vi "distribute_equally.vi"(8 "error in (no error)":errorcluster, 11 "TrajectoryDL091126GenericVoxel in":refnum<class "TrajectoryDL091126GenericVoxel.lvclass">) -> (0 "error out":errorcluster, 2 "failed?":bool, 3 "TrajectoryDL091126GenericVoxel out":refnum<class "TrajectoryDL091126GenericVoxel.lvclass">)   [LabVIEW 2010, in "TrajectoryDL091126GenericVoxel.lvclass"]
uses:
  TrajectoryDL091126GenericVoxel.lvclass
  common/classes/SpaceVector/SpaceVector/SpaceVector.lvclass
  common/classes/ErrorController/ErrorController/class_data.vi
  common/classes/ErrorController/ErrorController/ErrorController.lvclass
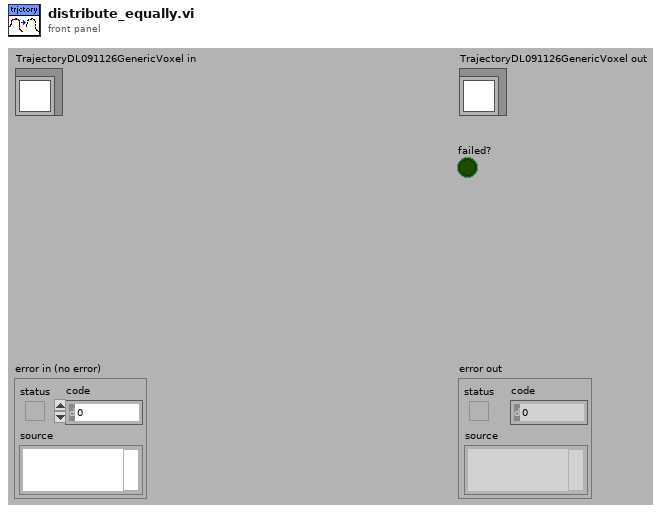
[diagram p1: front panel]
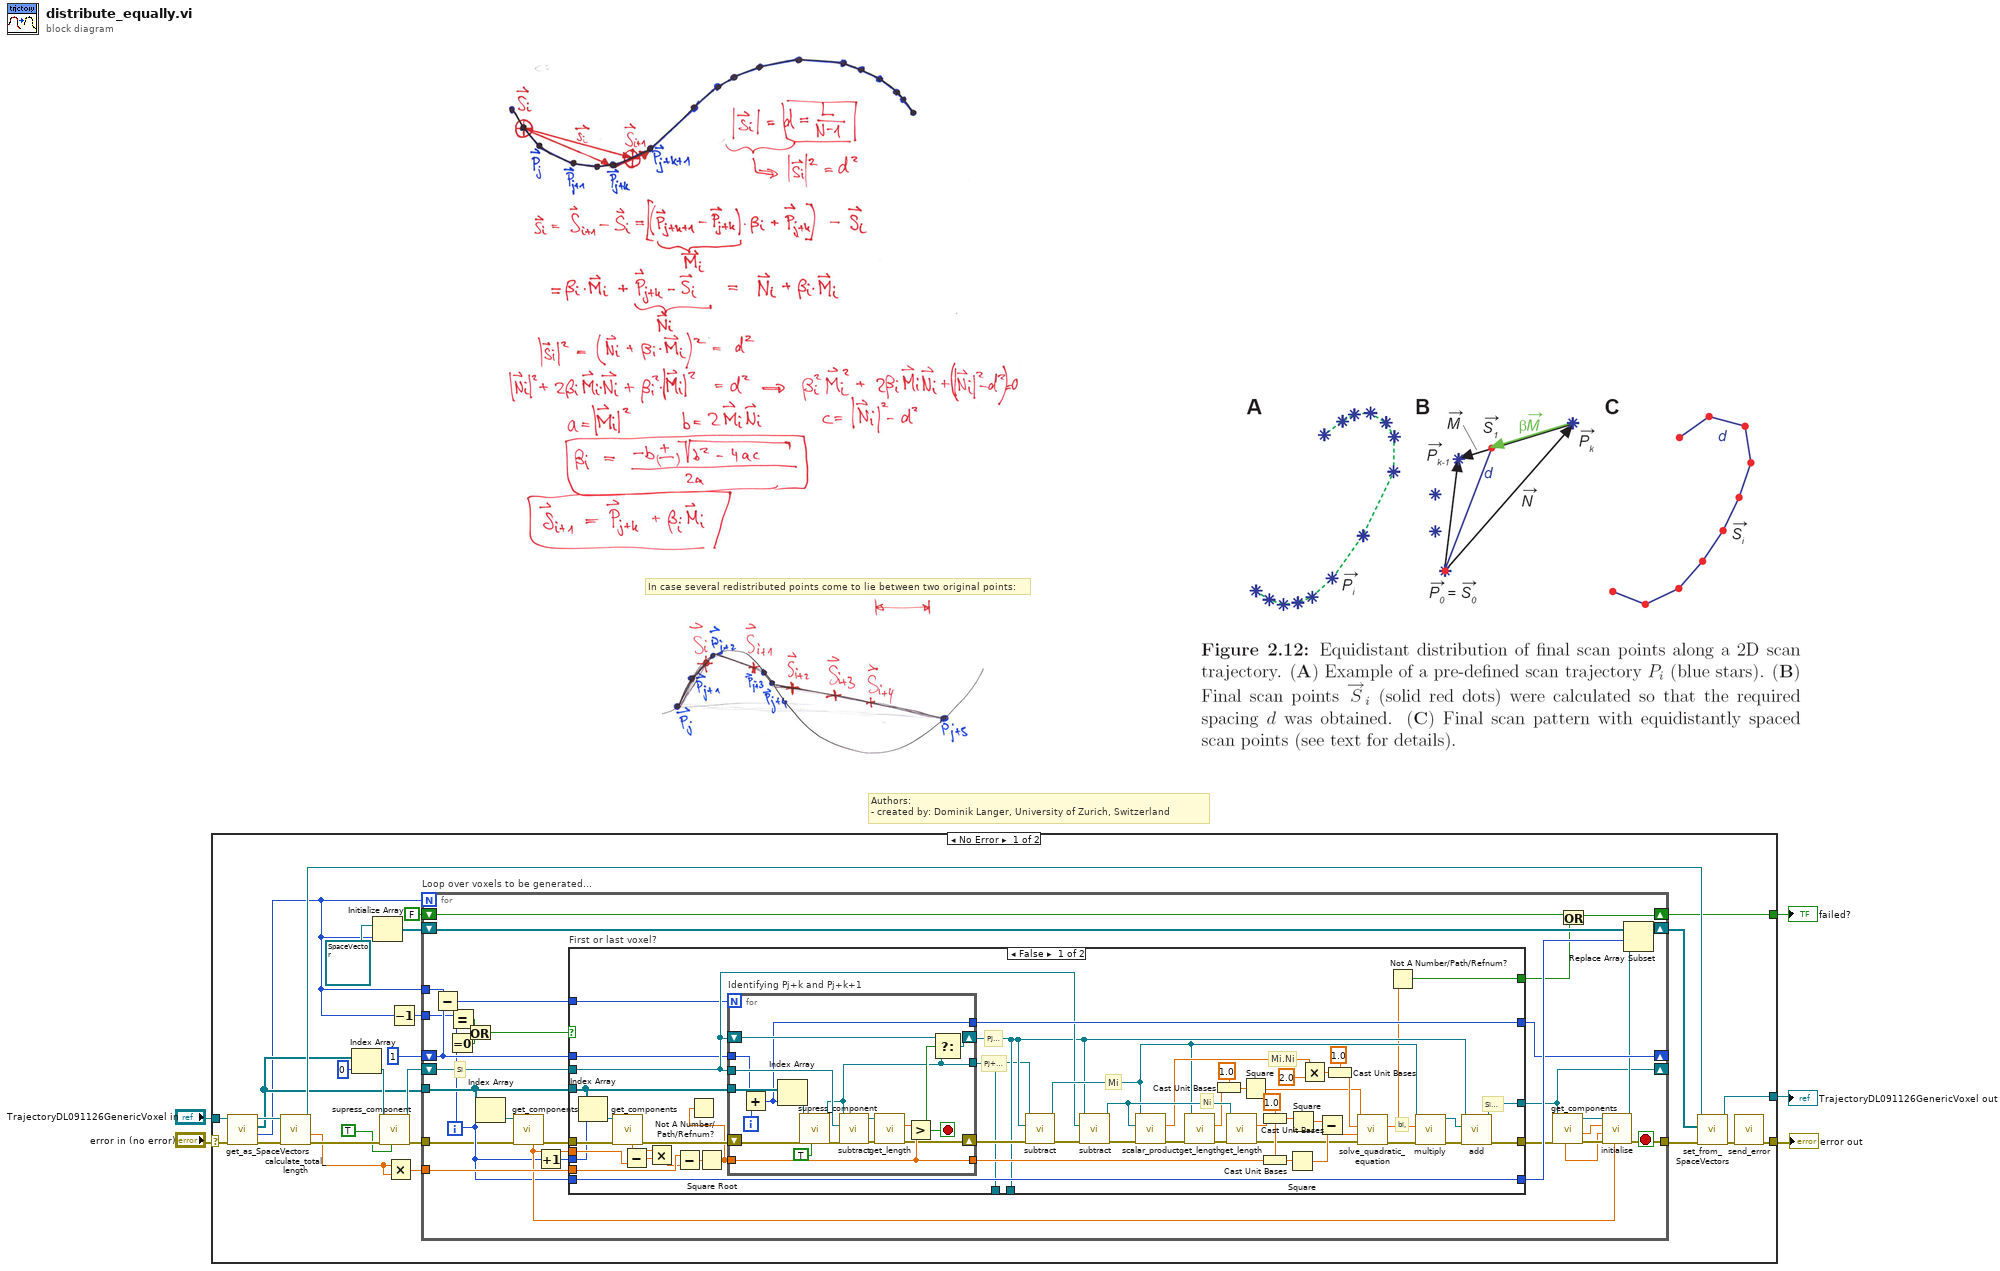
[diagram p0: block diagram]
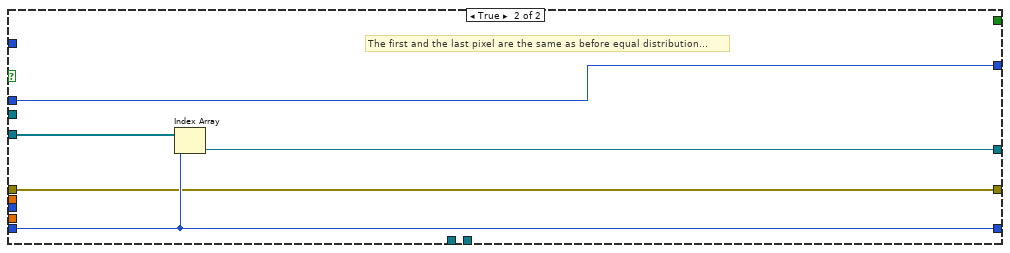
[diagram p2: hidden frame]
diagram:
  # "In case several redistributed points come to lie between two original points:"
  # "Authors: \n- created by: Dominik Langer, University of Zurich, Switzerland"
  n1 = case shown="No Error" "error in (no error)" {
    selector: "error in (no error)" -> [w27 w138]
    tunnel: [w6 w138] -> w4
    tunnel: [w23 w137] -> w2
    tunnel: "TrajectoryDL091126GenericVoxel in" -> [w26 w137]
    tunnel: [w8 _] -> w1
    frame No Error {
      n2 = call-dynamic "get_as_SpaceVectors.vi"("error in (no error)"=w27, "TrajectoryDL091126GenericVoxel in"=w26) -> ("error out"=w25:errorcluster, "number of voxels"=w11:i32, "voxels"=w12:refnum<class "SpaceVector.lvclass">[], "TrajectoryDL091126GenericVoxel out"=w24:refnum<class "TrajectoryDL091126GenericVoxel.lvclass">)  [unwired: 6 in]
      n3 = call-dynamic "calculate_total_length.vi"("error in (no error)"=w25, "TrajectoryDL091126GenericVoxel in"=w24) -> ("error out"=w19:errorcluster, "inter-pixel distance"=w13:dbl[unit], "TrajectoryDL091126GenericVoxel out"=w22:refnum<class "TrajectoryDL091126GenericVoxel.lvclass">)  [unwired: 6 in, 1 out]
      n4 = Index Array(array=w12, index=0) -> (element=w17:refnum<class "SpaceVector.lvclass">)
      n5 = Initialize Array(refnum<class "SpaceVector.lvclass"> refnum ("SpaceVector.lvclass"), w11) -> (w31:refnum<class "SpaceVector.lvclass">[])
      n6 = call "supress_component.vi"("z"=TRUE, "error in (no error)"=w19, "SpaceVector in"=w17) -> ("error out"=w18:errorcluster, "SpaceVector out"=w16:refnum<class "SpaceVector.lvclass">)  [unwired: 7 in]
      n7 = Multiply(x=w13, y=w13) -> (x*y=w14:dbl[unit])
      n8 = Decrement(x=w11) -> (x-1=w29:i32)
      n9 = for "Loop over voxels to be generated..." {
        N: w11 -> [_]
        tunnel: w12 -> [w39]
        tunnel: w14 -> [w43]
        shift-right: [w61] -> w21
        shift-left: w31 -> [w62]
        tunnel: w29 -> [w53]
        shift-right: [w56] -> _
        shift-left: 1 -> [w55]
        shift-right: [w44] -> _
        shift-left: w16 -> [w38]
        tunnel: w11 -> [w54]
        shift-right: [w33] -> w8
        shift-left: FALSE -> [w35]
        tunnel: w18 -> [w36]
        tunnel: [w32] -> w10
        i -> [w37]
        stop <- w32 stop-if-true
        # "Si"
        n10 = Subtract(x=w54, y=w55) -> (x-y=w52:i32)
        n11 = Equal To 0?(x=w37) -> (x = 0?=w58:bool)
        n12 = Equal?(x=w53, y=w37) -> (x = y?=w59:bool)
        n13 = Or(x=w59, y=w58) -> (x .or. y?=w57:bool)
        n14 = Index Array(array=w39, index=w37) -> (element=w51:refnum<class "SpaceVector.lvclass">)
        n15 = call "get_components.vi"("error in (no error)"=w36, "SpaceVector in"=w51) -> ("error out"=w41:errorcluster, "z"=w42:dbl[unit])  [unwired: 4 in, 4 out]
        n16 = Increment(x=w37) -> (x+1=w40:i32)
        n17 = case "First or last voxel?" shown="False" w57 {
          tunnel: w39 -> [w76 w136]
          tunnel: [w87 w132] -> w50
          tunnel: w41 -> [w75 w132]
          tunnel: [w86 w133] -> w44
          tunnel: w52 -> [w80 _]
          tunnel: [w108 w134] -> w60
          tunnel: w55 -> [w79 w135]
          tunnel: [w109 w135] -> w56
          tunnel: w37 -> [w108 w134]
          tunnel: w38 -> [w82 _]
          tunnel: w43 -> [w73 _]
          tunnel: w42 -> [w70 _]
          tunnel: w40 -> [w68 _]
          tunnel: [w66 _] -> _
          tunnel: [w65 _] -> _
          tunnel: [w63 _] -> w34
          frame False {
            w99 = 1.0 ("unit (none)")
            # "Ni"
            # "Mi"
            # "Pj+k+1"
            # "Pj+k"
            # "Si+1,x"
            # "bi,"
            # "Mi.Ni"
            n18 = Index Array(array=w76, index=w68) -> (element=w78:refnum<class "SpaceVector.lvclass">)
            n19 = call "get_components.vi"("error in (no error)"=w75, "SpaceVector in"=w78) -> ("error out"=w77:errorcluster, "z"=w71:dbl[unit])  [unwired: 4 in, 4 out]
            n20 = Subtract(x=w71, y=w70) -> (x-y=w69:dbl[unit])
            n21 = Multiply(x=w69, y=w69) -> (x*y=w72:dbl[unit])
            n22 = Subtract(x=w73, y=w72) -> (x-y=w74:dbl[unit])
            n23 = Square Root(x=w74) -> (sqrt(x)=w67:dbl[unit])
            n24 = Not A Number/Path/Refnum?(number/path/refnum=w67) -> ()  [unwired: 1 out]
            n25 = for "Identifying Pj+k and Pj+k+1" {
              N: w80 -> [_]
              tunnel: w76 -> [w131]
              tunnel: w79 -> [w115]
              tunnel: w67 -> [w127]
              shift-right: [w130] -> w66
              shift-left: w82 -> [w129]
              tunnel: [w116] -> w65
              tunnel: [w127] -> w100
              tunnel: [w121] -> w109
              shift-right: [w125] -> w107
              shift-left: w77 -> [w120]
              tunnel: w82 -> [w122]
              i -> [w114]
              stop <- w128 stop-if-true
              n26 = Add(x=w115, y=w114) -> (x+y=w121:i32)
              n27 = Index Array(array=w131, index=w121) -> (element=w117:refnum<class "SpaceVector.lvclass">)
              n28 = call "supress_component.vi"("z"=TRUE, "error in (no error)"=w120, "SpaceVector in"=w117) -> ("error out"=w119:errorcluster, "SpaceVector out"=w116:refnum<class "SpaceVector.lvclass">)  [unwired: 7 in]
              n29 = call "subtract.vi"("error in (no error)"=w119, "subtrahend"=w122, "SpaceVector in"=w116) -> ("error out"=w126:errorcluster, "SpaceVector out"=w124:refnum<class "SpaceVector.lvclass">)  [unwired: 7 in]
              n30 = call "get_length.vi"("error in (no error)"=w126, "SpaceVector in"=w124) -> ("error out"=w125:errorcluster, "length"=w123:dbl[unit])  [unwired: 7 in, 1 out]
              n31 = Greater?(x=w123, y=w127) -> (0:w128:bool)
              n32 = Select(t=w129, s=w128, f=w116) -> (s? t:f=w130:refnum<class "SpaceVector.lvclass">)
            }
            n33 = call "subtract.vi"("error in (no error)"=w107, "subtrahend"=w66, "SpaceVector in"=w65) -> ("error out"=w106:errorcluster, "SpaceVector out"=w83:refnum<class "SpaceVector.lvclass">)  [unwired: 7 in]
            n34 = call "subtract.vi"("error in (no error)"=w106, "subtrahend"=w82, "SpaceVector in"=w66) -> ("error out"=w95:errorcluster, "SpaceVector out"=w93:refnum<class "SpaceVector.lvclass">)  [unwired: 7 in]
            n35 = call "scalar_product.vi"("error in (no error)"=w95, "B in"=w93, "A in"=w83) -> ("error out"=w94:errorcluster, "scalar product"=w91:dbl[unit])  [unwired: 6 in, 1 out]
            n36 = call "get_length.vi"("error in (no error)"=w94, "SpaceVector in"=w83) -> ("error out"=w105:errorcluster, "length"=w84:dbl[unit])  [unwired: 7 in, 1 out]
            n37 = Cast Unit Bases(0:w84, 1:1.0 ("unit (none)")) -> (2:w104:dbl)
            n38 = call "get_length.vi"("error in (no error)"=w105, "SpaceVector in"=w93) -> ("error out"=w90:errorcluster, "length"=w81:dbl[unit])  [unwired: 7 in, 1 out]
            n39 = Square(x=w104) -> (x^2=w103:dbl)
            n40 = Cast Unit Bases(0:w81, 1:w99) -> (2:w102:dbl)
            n41 = Cast Unit Bases(0:w100, 1:w99) -> (2:w98:dbl)
            n42 = Square(x=w98) -> (x^2=w97:dbl)
            n43 = Square(x=w102) -> (x^2=w101:dbl)
            n44 = Multiply(x=w91, y=2.0) -> (x*y=w112:dbl[unit])
            n45 = Subtract(x=w101, y=w97) -> (x-y=w96:dbl)
            n46 = Cast Unit Bases(0:w112, 1:1.0 ("unit (none)")) -> (2:w110:dbl)
            n47 = call "solve_quadratic_equation.vi"("error in (no error)"=w90, "c"=w96, "b"=w110, "a"=w103) -> ("error out"=w89:errorcluster, "x1 (bigger result)"=w64:dbl)  [unwired: 5 in, 1 out]
            n48 = Not A Number/Path/Refnum?(number/path/refnum=w64) -> (NaN/Path/Refnum?=w63:bool)
            n49 = call "multiply.vi"("error in (no error)"=w89, "factor"=w64, "SpaceVector in"=w83) -> ("error out"=w88:errorcluster, "SpaceVector out"=w85:refnum<class "SpaceVector.lvclass">)  [unwired: 7 in]
            n50 = call "add.vi"("error in (no error)"=w88, "vector to be added"=w85, "SpaceVector in"=w66) -> ("error out"=w87:errorcluster, "SpaceVector out"=w86:refnum<class "SpaceVector.lvclass">)  [unwired: 7 in]
          }
          frame True {
            # "The first and the last pixel are the same as before equal distribution..."
            n51 = Index Array(array=w136, index=w134) -> (element=w133:refnum<class "SpaceVector.lvclass">)
          }
        }
        n52 = call "get_components.vi"("error in (no error)"=w50, "SpaceVector in"=w44) -> ("error out"=w49:errorcluster, "x"=w47:dbl[unit], "SpaceVector out"=w48:refnum<class "SpaceVector.lvclass">, "y"=w46:dbl[unit])  [unwired: 4 in, 2 out]
        n53 = Or(x=w35, y=w34) -> (x .or. y?=w33:bool)
        n54 = call "initialise.vi"("z"=w42, "error in (no error)"=w49, "y"=w46, "x"=w47, "SpaceVector in"=w48) -> ("error out"=w32:errorcluster, "SpaceVector out"=w45:refnum<class "SpaceVector.lvclass">)  [unwired: 5 in]
        n55 = Replace Array Subset(array=w62, new element=w45, index=w60) -> (w61:refnum<class "SpaceVector.lvclass">[])
      }
      n56 = call-dynamic "set_from_SpaceVectors.vi"("error in (no error)"=w10, "voxels"=w21, "TrajectoryDL091126GenericVoxel in"=w22) -> ("error out"=w7:errorcluster, "TrajectoryDL091126GenericVoxel out"=w23:refnum<class "TrajectoryDL091126GenericVoxel.lvclass">)  [unwired: 7 in]
      n57 = call "send_error.vi"("error in (no error)"=w7) -> ("error out"=w6:errorcluster)  [unwired: 10 in]
    }
    frame Error {
    }
  }
  "error out" <- w4
  "TrajectoryDL091126GenericVoxel out" <- w2
  "failed?" <- w1
